vi "Attenuator VNA Calibration Warning.vi"(4 "Current Stimulus":T5={"ATT Stimulus"={"Normalize"=TRUE, "Value (dB)"=0.0}, "VNA Stimulus"={"Use Instrument Settings"=FALSE, "Blank Frequencies"=FALSE, "Sweep Type"=enum."Linear", "Sweep"={"Fstart"=500.0, "Fstop"=1500.0, "Units"=enum."MHz", "Points"=201}, "Power (dBm)"=999.0, "IFBW (Hz)"=-1.0, "Sweep Time (s)"=-1.0, "Calibration"={"State"=FALSE, "String"=""}}} {"VNA Stimulus"."Sweep Time (s)" format="%.3g"}, 6 "Requested Stimulus":T5={"ATT Stimulus"={"Normalize"=TRUE, "Value (dB)"=0.0}, "VNA Stimulus"={"Use Instrument Settings"=FALSE, "Blank Frequencies"=FALSE, "Sweep Type"=enum."Linear", "Sweep"={"Fstart"=500.0, "Fstop"=1500.0, "Units"=enum."MHz", "Points"=201}, "Power (dBm)"=999.0, "IFBW (Hz)"=-1.0, "Sweep Time (s)"=-1.0, "Calibration"={"State"=FALSE, "String"=""}}} {"VNA Stimulus"."Sweep Time (s)" format="%.3g"}, 7 "Current Parameters to Measure":T1[](array[typedef]) {"Channel" min=1 max=99 step=1; "Parameter"."Stimulus Port" min=1 step=1; "Parameter"."Response Port" min=1 step=1}, 8 "error in (no error)":errorcluster, 9 "Parameters to Measure":T1[](array[typedef]) {"Channel" min=1 max=99 step=1; "Parameter"."Stimulus Port" min=1 step=1; "Parameter"."Response Port" min=1 step=1}, 11 "Message (\"\")":string="The instrument does not have a calibration state consistent\nwith the measurements to be performed.  Spartan always\nrecords the instrument calibration state when test sequences\nare executed.\n\nPlease select one of the following options:\n\n    Calibrate  -  run a calibration on the instrument now\n    Restore  -  restore a calibrated instrument state\n    Ignore  -  continue without calibration\n    Abort  -  abort this test execution\n    Abort All  -  abort the entire sequence") -> (0 "error out":errorcluster, 3 "Choice":T9=enum."Restore")   [LabVIEW 2011]
uses:
  TypeDefs/Attenuator Dialog Response.ctl
  TypeDefs/Attenuator Parameter to Measure.ctl
  S Parameter/TypeDefs/SP Parameter.ctl
  TypeDefs/Attenuator VNA Calibration State.ctl
  S Parameter/TypeDefs/SP Measurement Format.ctl
  TypeDefs/Attenuator Stimulus Parameters.ctl
  TypeDefs/Attenuator ATT Stimulus.ctl
  TypeDefs/Attenuator VNA Stimulus.ctl
  S Parameter/TypeDefs/SP Frequency Units.ctl
panel:
  in  "Abort All":bool
  in  "Abort":bool
  in  "Ignore":bool
  in  "Restore":bool
  in  "Calibrate":bool
  out "Current Cal":string
  out "Cur. Sweep Time":string="0.000"
  out "Req. Sweep Time":string="0.000" caption="Sweep Time"
  out "Sweep Time":cluster{"Pass":bool, "Fail":bool}={"Pass"=TRUE, "Fail"=FALSE}
  out "Cur. IFBW":string="0"
  out "Req. IFBW":string="0" caption="IFBW"
  out "IFBW":cluster{"Pass":bool, "Fail":bool}={"Pass"=TRUE, "Fail"=FALSE}
  out "Cur. Power":string="0"
  out "Req. Power":string="0" caption="Power"
  out "Power":cluster{"Pass":bool, "Fail":bool}={"Pass"=TRUE, "Fail"=FALSE}
  out "Cur. Points":string="0"
  out "Req. Points":string="0" caption="Number of Points"
  out "Points":cluster{"Pass":bool, "Fail":bool}={"Pass"=TRUE, "Fail"=FALSE}
  out "Cur. Stop Freq.":string="0.000"
  out "Req. Stop Freq.":string="0.000" caption="Stop Frequency"
  out "Stop Freq":cluster{"Pass":bool, "Fail":bool}={"Pass"=TRUE, "Fail"=FALSE}
  out "Cur. Start Freq.":string="0.000"
  out "Req. Start Freq.":string="0.000" caption="Start Fequency"
  out "Start Freq":cluster{"Pass":bool, "Fail":bool}={"Pass"=TRUE, "Fail"=FALSE}
  out "Cur. Sweep Type":string="Linear"
  out "Req. Sweep Type":string="Linear" caption="Sweep Type"
  out "Sweep Type":cluster{"Pass":bool, "Fail":bool}={"Pass"=TRUE, "Fail"=FALSE}
  # "Requested"
  # "Current"
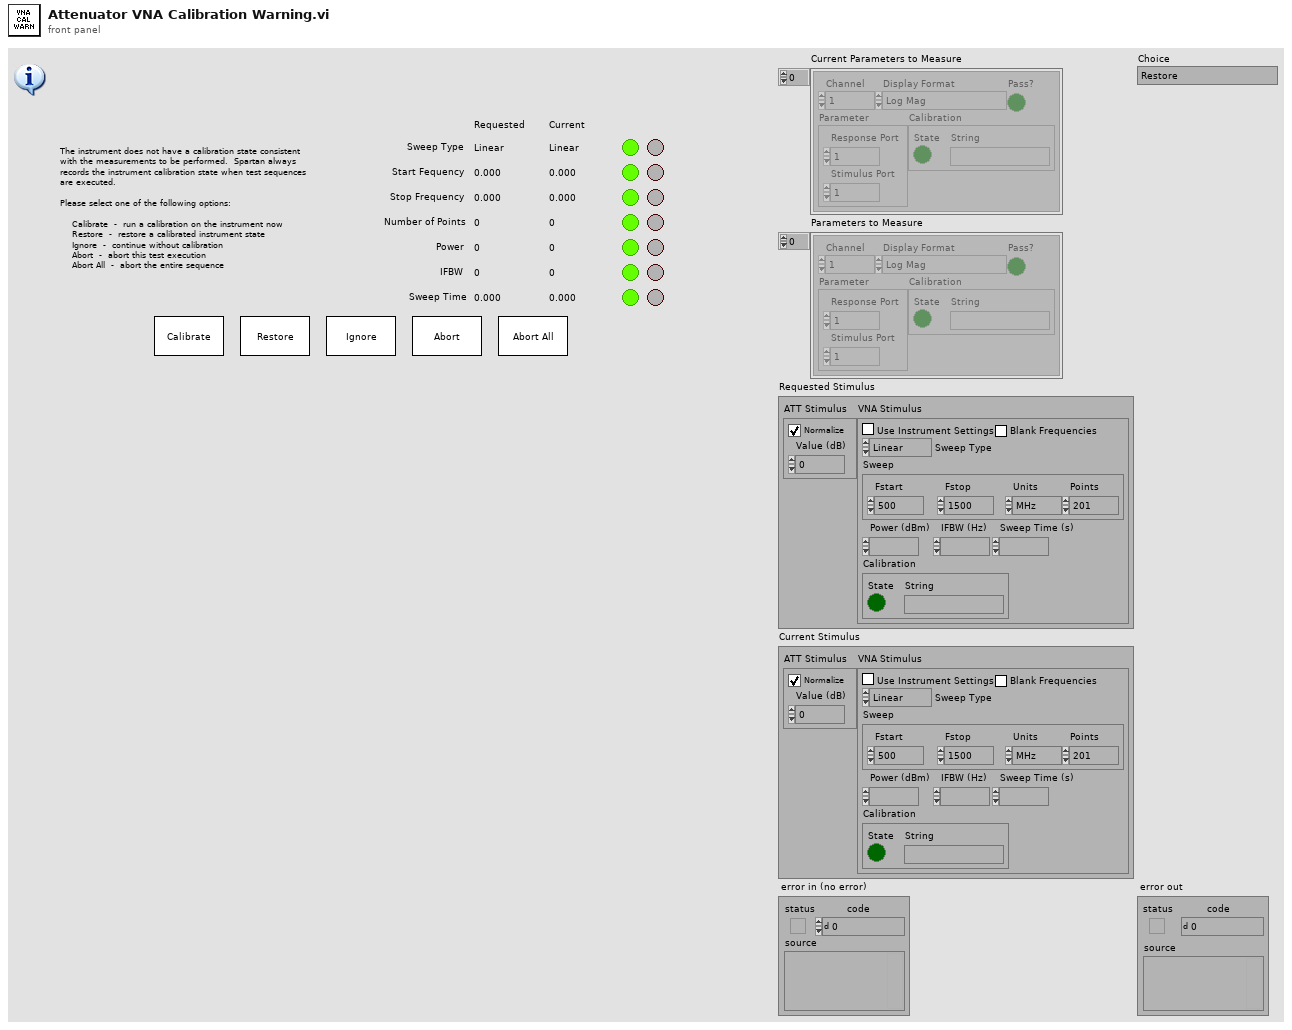
[diagram p1: front panel]
types:
  T1 = typedef "Attenuator Parameter to Measure.ctl" = cluster{"Channel":i8, "Parameter":T2, "Calibration":T3, "Display Format":T4, "Pass?":bool}
  T2 = typedef "SP Parameter.ctl" = cluster{"Stimulus Port":i8, "Response Port":i8}
  T3 = typedef "Attenuator VNA Calibration State.ctl" = cluster{"State":bool, "String":string}
  T4 = typedef "SP Measurement Format.ctl" = enum32{"Log Mag", "Phase", "Delay", "Smith (R+jX)", "Polar (Re/Im)", "Linear Mag", "SWR", "Real", "Imaginary", "Smith (Lin/Phase)", "Smith (Log/Phase)", "Smith (Real/Imag)", "Smith (G+jB)", "Polar (Lin/Phase)", "Polar (Log/Phase)", "Expanded Phase", "Positive Phase", "Inverted Smith", "Unwrapped Phase", "Power Out", "Power In", "Linear Mag/Phase", "Log Mag/Phase", "Real/Imaginary"}
  T5 = typedef "Attenuator Stimulus Parameters.ctl" = cluster{"ATT Stimulus":T6, "VNA Stimulus":T7}
  T6 = typedef "Attenuator ATT Stimulus.ctl" = cluster{"Normalize":bool, "Value (dB)":dbl}
  T7 = typedef "Attenuator VNA Stimulus.ctl" = cluster{"Use Instrument Settings":bool, "Blank Frequencies":bool, "Sweep Type":enum32{"Linear", "Logarithmic", "List", "Power", "CW"}, "Sweep":cluster{"Fstart":dbl, "Fstop":dbl, "Units":T8, "Points":i32}, "Power (dBm)":dbl, "IFBW (Hz)":dbl, "Sweep Time (s)":dbl, "Calibration":T3}
  T8 = typedef "SP Frequency Units.ctl" = enum16{"Hz", "kHz", "MHz", "GHz", "Points"}
  T9 = typedef "Attenuator Dialog Response.ctl" = enum16{"None", "Calibrate", "Restore", "Ignore", "Abort", "Abort All"}
  T10 = enum32{"Linear", "Logarithmic", "List", "Power", "CW"}
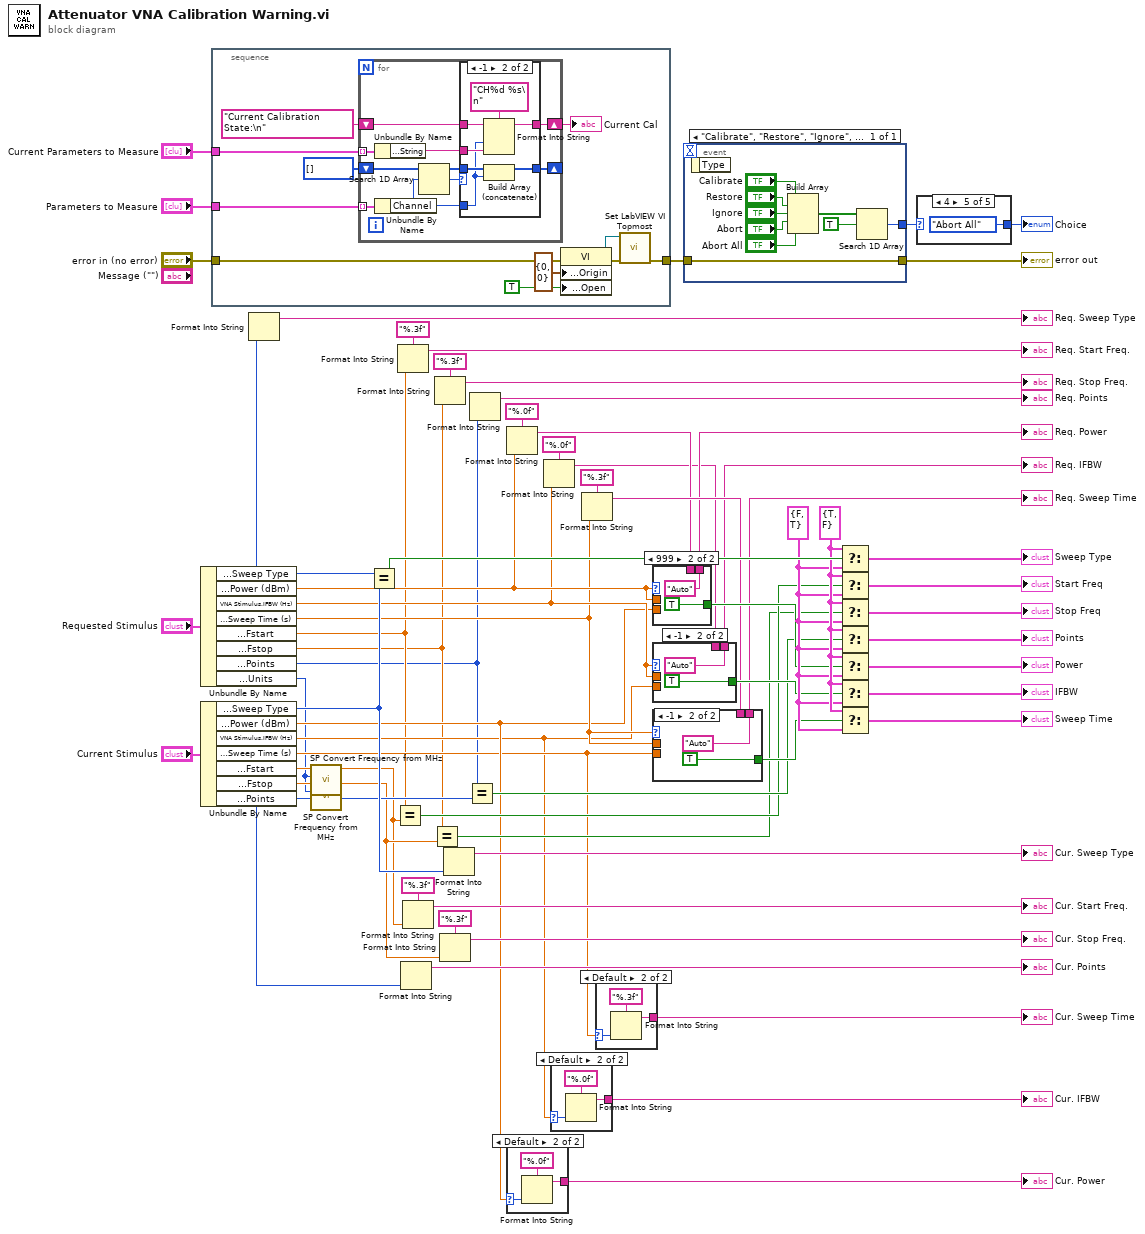
[diagram p0: block diagram]
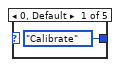
[diagram p2: hidden frame]
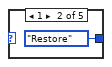
[diagram p3: hidden frame]
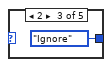
[diagram p4: hidden frame]
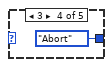
[diagram p5: hidden frame]
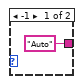
[diagram p6: hidden frame]
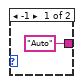
[diagram p7: hidden frame]
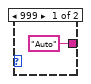
[diagram p8: hidden frame]
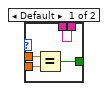
[diagram p9: hidden frame]
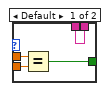
[diagram p10: hidden frame]
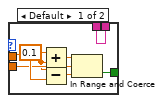
[diagram p11: hidden frame]
diagram:
  w47 = cluster{"Pass":bool, "Fail":bool} {"Pass"=FALSE, "Fail"=TRUE} ("Sweep Type")
  w48 = cluster{"Pass":bool, "Fail":bool} {"Pass"=TRUE, "Fail"=FALSE} ("Sweep Type")
  n1 = Unbundle By Name("Requested Stimulus") -> ("VNA Stimulus.Sweep Type"=w59:T10, "VNA Stimulus.Power (dBm)"=w34:dbl, "VNA Stimulus.IFBW (Hz)"=w32:dbl, "VNA Stimulus.Sweep Time (s)"=w30:dbl, "VNA Stimulus.Sweep.Fstart"=w10:dbl, "VNA Stimulus.Sweep.Fstop"=w9:dbl, "VNA Stimulus.Sweep.Points"=w8:i32, "VNA Stimulus.Sweep.Units"=w3:T8)
  n2 = Unbundle By Name("Current Stimulus") -> ("VNA Stimulus.Sweep Type"=w56:T10, "VNA Stimulus.Power (dBm)"=w16:dbl, "VNA Stimulus.IFBW (Hz)"=w12:dbl, "VNA Stimulus.Sweep Time (s)"=w15:dbl, "VNA Stimulus.Sweep.Fstart"=w7:dbl, "VNA Stimulus.Sweep.Fstop"=w6:dbl, "VNA Stimulus.Sweep.Points"=w11:i32)
  n3 = stacked-sequence {
    tunnel: "error in (no error)" -> [w77]
    tunnel: [w73] -> w63
    tunnel: "Parameters to Measure" -> [w75]
    tunnel: "Current Parameters to Measure" -> [w68]
    frame #0 {
      n4 = for {
        tunnel: w75 -> [w86] mode=indexing
        shift-right: [w83] -> w69
        shift-left: "Current Calibration State:\n" -> [w84]
        tunnel: w68 -> [w82] mode=indexing
        shift-right: [w78] -> _
        shift-left: i8[] [] -> [w79]
        n5 = Unbundle By Name(w82) -> ("Calibration.String"=w85:string)
        n6 = Unbundle By Name(w86) -> ("Channel"=w81:i8)
        n7 = Search 1D Array(1D array=w79, element=w81) -> (index of element=w80:i32)  [unwired: 1 out]
        n8 = case shown="-1" w80 {
          tunnel: w85 -> [_ w95]
          tunnel: w84 -> [w88 w93]
          tunnel: [w88 w92] -> w83
          tunnel: w81 -> [_ w89]
          tunnel: w79 -> [w87 w91]
          tunnel: [w87 w90] -> w78
          frame Default {
          }
          frame -1 {
            n9 = Format Into String(format string="CH%d %s\n", initial string=w93, w89, w95) -> (resulting string=w92:string)  [unwired: 1 in, 1 out]
            n10 = Build Array (concatenate)(w91, w89) -> (w90:i8[])
          }
        }
      }
      "Current Cal" <- w69
      n11 = property on="Property Node" class="VI"(error in=w77, "Front Panel Window:Origin"=cluster{"Horizontal":i16, "Vertical":i16} {"Horizontal"=0, "Vertical"=0}, "Front Panel Window:Open"=TRUE) -> (reference out=w72:refnum<vi>, error out=w74:errorcluster)  [unwired: 1 in]
      n12 = call "Set LabVIEW VI Topmost.vi"("error in (no error)"=w74, "VI Refnum (null)"=w72) -> ("error out"=w73:errorcluster)  [unwired: 7 in, 2 out]
    }
  }
  n13 = Format Into String(w59) -> (resulting string=→"Req. Sweep Type":string)  [unwired: 3 in, 1 out]
  n14 = call "SP Convert Frequency from MHz.vi"("Units"=w3, "Frequency (MHz)"=w7) -> ("Converted Frequency"=w4:dbl)  [unwired: 1 in, 8 out]
  n15 = call "SP Convert Frequency from MHz.vi"("Units"=w3, "Frequency (MHz)"=w6) -> ("Converted Frequency"=w5:dbl)  [unwired: 1 in, 8 out]
  n16 = Equal?(x=w59, y=w56) -> (x = y?=w58:bool)
  n17 = Equal?(x=w10, y=w4) -> (x = y?=w42:bool)
  n18 = Format Into String(format string="%.3f", w10) -> (resulting string=→"Req. Start Freq.":string)  [unwired: 2 in, 1 out]
  n19 = Format Into String(w11) -> (resulting string=→"Cur. Points":string)  [unwired: 3 in, 1 out]
  n20 = Format Into String(format string="%.3f", w4) -> (resulting string=→"Cur. Start Freq.":string)  [unwired: 2 in, 1 out]
  n21 = Equal?(x=w9, y=w5) -> (x = y?=w41:bool)
  n22 = Format Into String(format string="%.3f", w9) -> (resulting string=→"Req. Stop Freq.":string)  [unwired: 2 in, 1 out]
  n23 = Format Into String(format string="%.3f", w5) -> (resulting string=→"Cur. Stop Freq.":string)  [unwired: 2 in, 1 out]
  n24 = Format Into String(w56) -> (resulting string=→"Cur. Sweep Type":string)  [unwired: 3 in, 1 out]
  n25 = Equal?(x=w8, y=w11) -> (x = y?=w43:bool)
  n26 = Format Into String(w8) -> (resulting string=→"Req. Points":string)  [unwired: 3 in, 1 out]
  n27 = Format Into String(format string="%.0f", w34) -> (resulting string=w21:string)  [unwired: 2 in, 1 out]
  n28 = case shown="Default" w16 {
    selector: w16 -> [_ w97]
    tunnel: ["Auto" w98] -> w24
    frame 999 {
    }
    frame Default {
      n29 = Format Into String(format string="%.0f", w97) -> (resulting string=w98:string)  [unwired: 2 in, 1 out]
    }
  }
  "Cur. Power" <- w24
  n30 = Format Into String(format string="%.0f", w32) -> (resulting string=w19:string)  [unwired: 2 in, 1 out]
  n31 = case shown="Default" w12 {
    selector: w12 -> [_ w101]
    tunnel: ["Auto" w102] -> w13
    frame -1 {
    }
    frame Default {
      n32 = Format Into String(format string="%.0f", w101) -> (resulting string=w102:string)  [unwired: 2 in, 1 out]
    }
  }
  "Cur. IFBW" <- w13
  n33 = Format Into String(format string="%.3f", w30) -> (resulting string=w23:string)  [unwired: 2 in, 1 out]
  n34 = case shown="Default" w15 {
    selector: w15 -> [_ w105]
    tunnel: ["Auto" w106] -> w14
    frame -1 {
    }
    frame Default {
      n35 = Format Into String(format string="%.3f", w105) -> (resulting string=w106:string)  [unwired: 2 in, 1 out]
    }
  }
  "Cur. Sweep Time" <- w14
  n36 = case shown="999" w34 {
    tunnel: w34 -> [w111 _]
    tunnel: w16 -> [w110 _]
    tunnel: [w109 TRUE] -> w46
    tunnel: w21 -> [w108 _]
    tunnel: [w108 "Auto" ("format string")] -> w20
    frame Default {
      n37 = Equal?(x=w111, y=w110) -> (x = y?=w109:bool)
    }
    frame 999 {
    }
  }
  "Req. Power" <- w20
  n38 = case shown="-1" w32 {
    tunnel: w32 -> [w117 _]
    tunnel: w12 -> [w116 _]
    tunnel: [w115 TRUE] -> w45
    tunnel: w19 -> [w114 _]
    tunnel: [w114 "Auto" ("format string")] -> w18
    frame Default {
      n39 = Equal?(x=w117, y=w116) -> (x = y?=w115:bool)
    }
    frame -1 {
    }
  }
  "Req. IFBW" <- w18
  n40 = case shown="-1" w30 {
    tunnel: w30 -> [w120 _]
    tunnel: w15 -> [w121 _]
    tunnel: [w123 TRUE] -> w44
    tunnel: w23 -> [w122 _]
    tunnel: [w122 "Auto" ("format string")] -> w22
    frame Default {
      w124 = 0.1
      n41 = Add(x=w124, y=w120) -> (x+y=w126:dbl)
      n42 = Subtract(x=w120, y=w124) -> (x-y=w125:dbl)
      n43 = In Range and Coerce(upper limit=w126, x=w121, lower limit=w125) -> (In Range?=w123:bool)  [unwired: 1 out]
    }
    frame -1 {
    }
  }
  "Req. Sweep Time" <- w22
  n44 = event shown="[0] \"Calibrate\", \"Restore\", \"Ignore\", \"Abort\", \"Abort All\": Value Change" {
    selector: _ -> [_]
    dyn-events: _ -> [_]
    timeout: _ -> [_]
    tunnel: w63 -> [w137]
    tunnel: [w137] -> w66
    tunnel: [w130] -> w2
    event "Calibrate", "Restore", "Ignore", "Abort", "Abort All": Value Change {
      n45 = event-data() -> ()  [unwired: 2 out]
      n46 = Build Array("Calibrate", "Restore", "Ignore", "Abort", "Abort All") -> (w132:bool[])
      n47 = Search 1D Array(1D array=w132, element=TRUE) -> (index of element=w130:i32)  [unwired: 1 out]
    }
  }
  "error out" <- w66
  n48 = Select(t=w48, s=w58, f=w47) -> (s? t:f=→"Sweep Type":cluster{"Pass":bool, "Fail":bool})
  n49 = Select(t=w48, s=w42, f=w47) -> (s? t:f=→"Start Freq":cluster{"Pass":bool, "Fail":bool})
  n50 = Select(t=w48, s=w41, f=w47) -> (s? t:f=→"Stop Freq":cluster{"Pass":bool, "Fail":bool})
  n51 = Select(t=w48, s=w43, f=w47) -> (s? t:f=→"Points":cluster{"Pass":bool, "Fail":bool})
  n52 = Select(t=w48, s=w46, f=w47) -> (s? t:f=→"Power":cluster{"Pass":bool, "Fail":bool})
  n53 = Select(t=w48, s=w45, f=w47) -> (s? t:f=→"IFBW":cluster{"Pass":bool, "Fail":bool})
  n54 = Select(t=w48, s=w44, f=w47) -> (s? t:f=→"Sweep Time":cluster{"Pass":bool, "Fail":bool})
  n55 = case shown="4" w2 {
    tunnel: [Attenuator_Dialog_Response."Calibrate" ("Action") Attenuator_Dialog_Response."Restore" ("Action") Attenuator_Dialog_Response."Ignore" ("Action") Attenuator_Dialog_Response."Abort" ("Action") Attenuator_Dialog_Response."Abort All" ("Action")] -> w1
    frame 0, Default {
    }
    frame 1 {
    }
    frame 2 {
    }
    frame 3 {
    }
    frame 4 {
    }
  }
  "Choice" <- w1
